vi "Switch channel.vi"(8 "error in":errorcluster, 9 "Channel":i32, 10 "Acquisition cluster":T1={"Save path"=path "D:/DATA_2018", "t frame"=0, "bookmark #"=0, "Z-current"=0, "Channel"=0, "total t frames"=0, "Total bookmarks"=0, "Total z steps"=0, "Total channels"=0, "Gain 1"=100, "Gain 2"=100, "Gain 3"=100, "Gain 4"=100, "Exposure 1"=100.0, "Exposure 2"=100.0, "Exposure 3"=100.0, "Exposure 4"=100.0, "Channel 1"="Red", "Channel 2"="None", "Channel 3"="None", "Channel 4"="None", "Bookmarks?"=FALSE, "Acquisition order"=enum."C-T-Z-B", "t-delay"=0.0, "z-step"=1.0, "Total Images"=1, "Start position"=[], "Piezo radio"=enum."Piezo off", "Piezo Step X"=20.0, "Piezo Step Y"=20.0, "Piezo Step Z"=20.0, "Piezo X current"=0.0, "Piezo Y current"=0.0, "Piezo Z current"=0.0, "LED illumination"=TRUE, "Piezo Amp X"=0.0, "Piezo Amp Y"=0.0, "Piezo Amp Z"=0.0}, 11 "Instrument cluster":T2) -> (0 "error out":errorcluster)   [LabVIEW 2017]
uses:
  C:/Program Files/National Instruments/LabVIEW 2017/instr.lib/IDS/ueye.NET/uEyeDotNet.dll
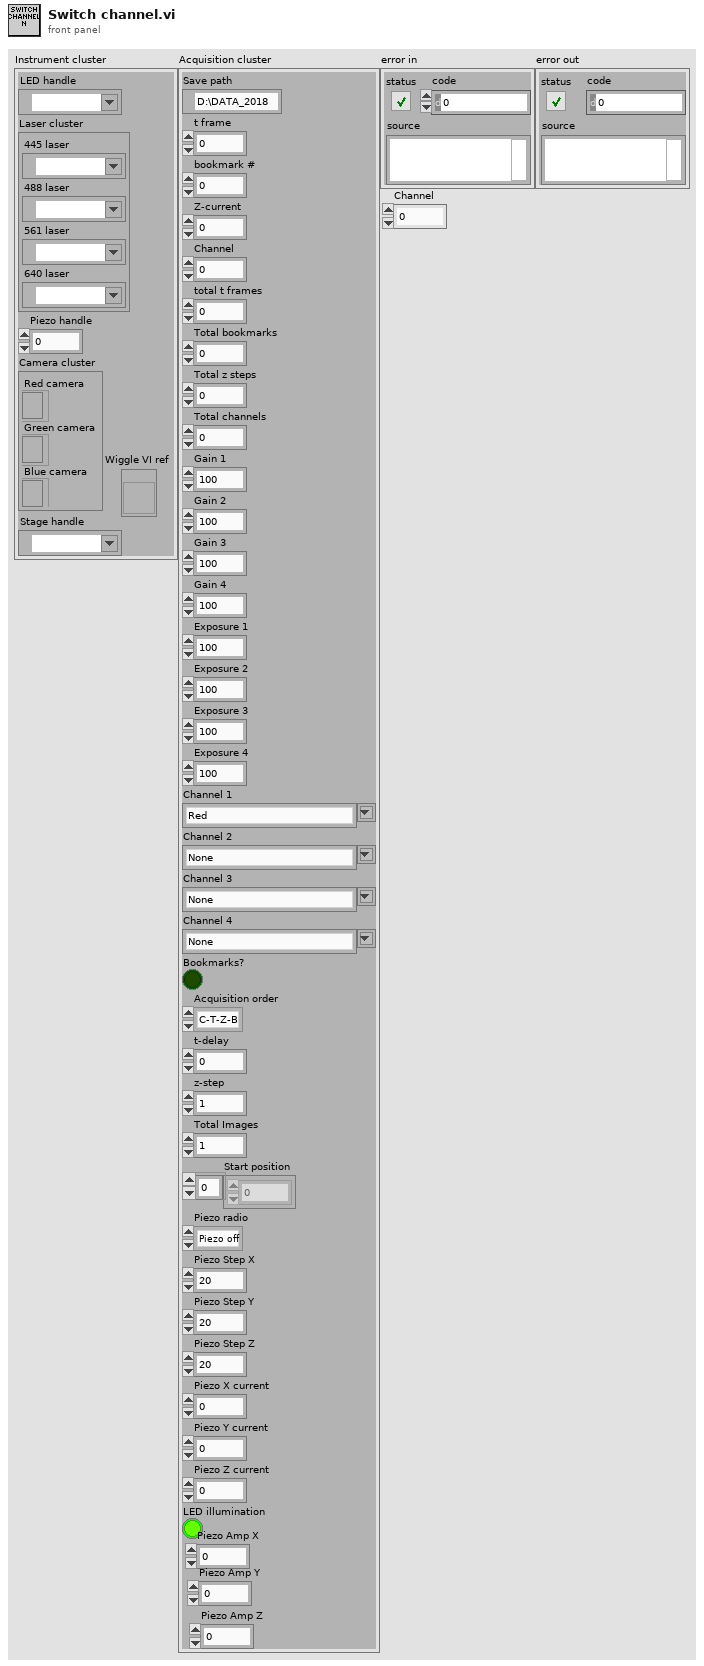
[diagram p1: front panel]
types:
  T1 = cluster{"Save path":path, "t frame":i32, "bookmark #":i32, "Z-current":i32, "Channel":i32, "total t frames":i32, "Total bookmarks":i32, "Total z steps":i32, "Total channels":i32, "Gain 1":i32, "Gain 2":i32, "Gain 3":i32, "Gain 4":i32, "Exposure 1":dbl, "Exposure 2":dbl, "Exposure 3":dbl, "Exposure 4":dbl, "Channel 1":string, "Channel 2":string, "Channel 3":string, "Channel 4":string, "Bookmarks?":bool, "Acquisition order":enum16{"C-T-Z-B", "C-T-B-Z", "C-Z-T-B", "C-Z-B-T", "C-B-T-Z", "C-B-Z-T", "T-C-Z-B", "T-C-B-Z", "T-Z-C-B", "T-Z-B-C", "T-B-C-Z", "T-B-Z-C", "Z-C-T-B", "Z-C-B-T", "Z-T-C-B", "Z-T-B-C", "Z-B-C-T", "Z-B-T-C", "B-C-T-Z", "B-C-Z-T", "B-Z-C-T", "B-Z-T-C", "B-T-C-Z", "B-T-Z-C"}, "t-delay":dbl, "z-step":dbl, "Total Images":i32, "Start position":dbl[], "Piezo radio":enum32{"Piezo off", "Piezo wiggle", "Piezo step"}, "Piezo Step X":dbl, "Piezo Step Y":dbl, "Piezo Step Z":dbl, "Piezo X current":dbl, "Piezo Y current":dbl, "Piezo Z current":dbl, "LED illumination":bool, "Piezo Amp X":dbl, "Piezo Amp Y":dbl, "Piezo Amp Z":dbl}
  T2 = cluster{"LED handle":refnum<visa-resource-name>, "Laser cluster":cluster{"445 laser":refnum<visa-resource-name>, "488 laser":refnum<visa-resource-name>, "561 laser":refnum<visa-resource-name>, "640 laser":refnum<visa-resource-name>}, "Piezo handle":i32, "Camera cluster":cluster{"Red camera":refnum<k24>, "Green camera":refnum<k24>, "Blue camera":refnum<k24>}, "Stage handle":refnum<visa-resource-name>, "Wiggle VI ref":refnum<vi>}
  T3 = cluster{"445 laser":refnum<visa-resource-name>, "488 laser":refnum<visa-resource-name>, "561 laser":refnum<visa-resource-name>, "640 laser":refnum<visa-resource-name>}
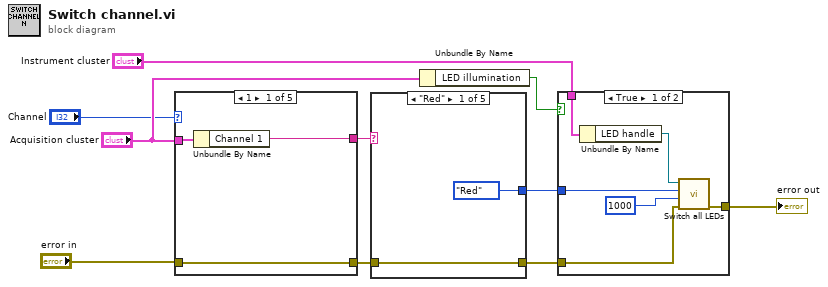
[diagram p0: block diagram]
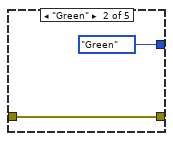
[diagram p2: hidden frame]
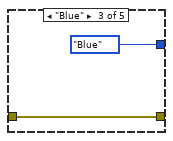
[diagram p3: hidden frame]
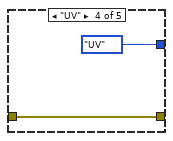
[diagram p4: hidden frame]
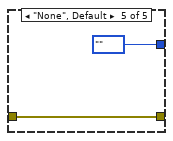
[diagram p5: hidden frame]
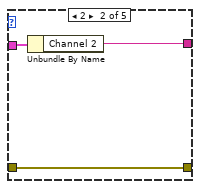
[diagram p6: hidden frame]
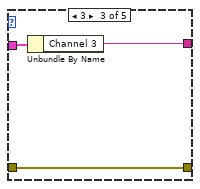
[diagram p7: hidden frame]
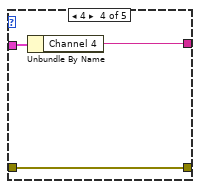
[diagram p8: hidden frame]
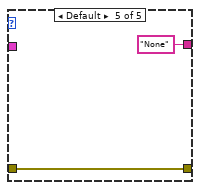
[diagram p9: hidden frame]
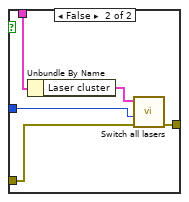
[diagram p10: hidden frame]
diagram:
  n1 = case shown="1" "Channel" {
    tunnel: "Acquisition cluster" -> [w13 w16 w19 w22 _]
    tunnel: "error in" -> [w11 w15 w18 w21 w23]
    tunnel: [w11 w15 w18 w21 w23] -> w2
    tunnel: [w12 w14 w17 w20 "None" ("Channel 4")] -> w10
    frame 1 {
      n2 = Unbundle By Name(w13) -> ("Channel 1"=w12:string)
    }
    frame 2 {
      n3 = Unbundle By Name(w16) -> ("Channel 2"=w14:string)
    }
    frame 3 {
      n4 = Unbundle By Name(w19) -> ("Channel 3"=w17:string)
    }
    frame 4 {
      n5 = Unbundle By Name(w22) -> ("Channel 4"=w20:string)
    }
    frame Default {
    }
  }
  n6 = case shown="\"Red\"" w10 {
    tunnel: [w25 w27 w29 w31 w34] -> w9
    tunnel: w2 -> [w25 w27 w29 w31 w34]
    tunnel: [enum8{"Red", "Green", "Blue", "UV", ""}."Red" ("Live channel") enum8{"Red", "Green", "Blue", "UV", ""}."Green" ("Live channel") enum8{"Red", "Green", "Blue", "UV", ""}."Blue" ("Live channel") enum8{"Red", "Green", "Blue", "UV", ""}."UV" ("Live channel") enum8{"Red", "Green", "Blue", "UV", ""}."" ("Live channel")] -> w8
    frame "Red" {
    }
    frame "Green" {
    }
    frame "Blue" {
    }
    frame "UV" {
    }
    frame "None", Default {
    }
  }
  n7 = Unbundle By Name("Acquisition cluster") -> ("LED illumination"=w3:bool)
  n8 = case shown="True" w3 {
    tunnel: w8 -> [w40 w43]
    tunnel: "Instrument cluster" -> [w39 w45]
    tunnel: w9 -> [w36 w42]
    tunnel: [w37 w41] -> w1
    frame True {
      n9 = Unbundle By Name(w39) -> ("LED handle"=w38:refnum<visa-resource-name>)
      n10 = call "Switch all LEDs.vi"("error in"=w36, "Switching delay (ms)"=u32 1000, "Live channel"=w40, "LED handle in"=w38) -> ("error out"=w37:errorcluster)  [unwired: 6 in, 1 out]
    }
    frame False {
      n11 = Unbundle By Name(w45) -> ("Laser cluster"=w44:T3)
      n12 = call "Switch all lasers.vi"("error in"=w42, "Live channel"=w43, "Laser cluster"=w44) -> ("error out"=w41:errorcluster)  [unwired: 8 in]
    }
  }
  "error out" <- w1
